vi "例8.11-1连续输出（非重复生成)2.vi"() -> ()   [LabVIEW 2017]
uses:
  <vilib>/measure/NI_MABase.lvlib
panel:
  in  "stop (F)":bool caption="停止(F)"
  in  "amplitude":dbl=1.0 caption="幅值" format="%0.2p"
  in  "frequency":dbl=10.0 caption="频率" format="%0.2p"
  out "波形图":waveform(dbl)(graph)
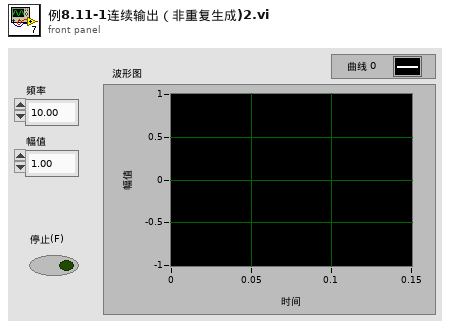
[diagram p1: front panel]
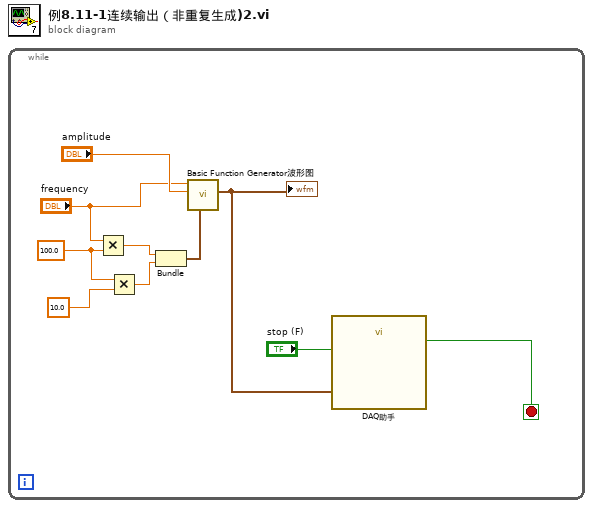
[diagram p0: block diagram]
diagram:
  n1 = while {
    stop <- w9 stop-if-true
    w5 = 100.0 ("y")
    n2 = Multiply(x="frequency", y=w5) -> (x*y=w3:dbl)
    n3 = Multiply(x=w5, y=10.0) -> (x*y=w2:dbl)
    n4 = Bundle(w3, w2) -> (w1:cluster{dbl, dbl})  [unwired: 1 in]
    n5 = call <vilib>:"Basic Function Generator.vi"("sampling info"=w1, "amplitude"="amplitude", "frequency"="frequency") -> ("signal out"=w7:waveform(dbl))  [unwired: 6 in, 2 out]
    "波形图" <- w7
    n6 = call "DAQ助手"("data"=w7, "stop (F)"="stop (F)") -> ("stopped"=w9:bool)  [unwired: 15 in, 2 out]
  }
